vi "Write StateUART.vi"(8 "error in (no error)":errorcluster, 10 "STATEUART":T1, 11 "GiaoTiepUART in":refnum<class "GiaoTiepUART.lvclass">) -> (0 "error out":errorcluster, 3 "GiaoTiepUART out":refnum<class "GiaoTiepUART.lvclass">)   [LabVIEW 2014, in "LibraryGcode.lvlib" / "GiaoTiepUART.lvclass"]
uses:
  GiaoTiepUART.lvclass
  StateMachine_UART.ctl
  GiaoTiepUART.lvclass/GiaoTiepUART.ctl
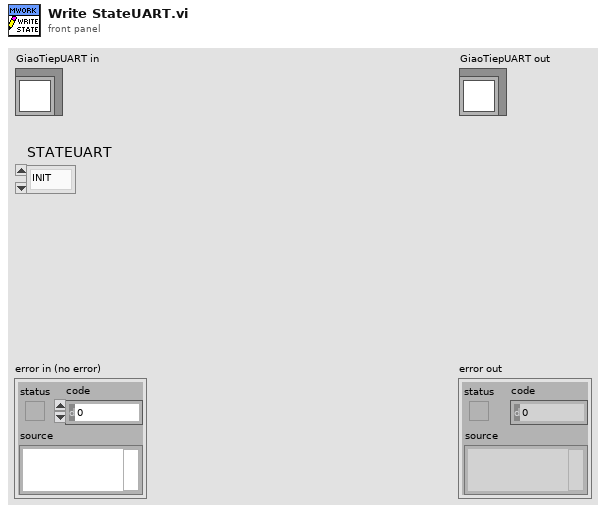
[diagram p1: front panel]
types:
  T1 = typedef "LibraryGcode.lvlib/GiaoTiepUART.lvclass/StateMachine_UART.ctl" = enum16{"INIT", "WRITE", "READ", "CHECKDATA", "IDLE", "STOP"}
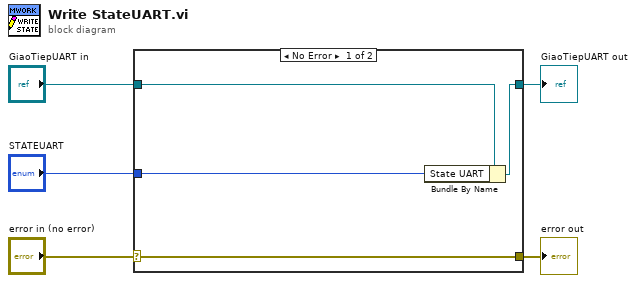
[diagram p0: block diagram]
diagram:
  n1 = case shown="No Error" "error in (no error)" {
    selector: "error in (no error)" -> [w9 w10]
    tunnel: [w9 w10] -> w4
    tunnel: [w8 w11] -> w2
    tunnel: "GiaoTiepUART in" -> [w6 w11]
    tunnel: "STATEUART" -> [w7 _]
    frame No Error {
      n2 = Bundle By Name(cluster=w6, "State UART"=w7) -> (w8:refnum<class "GiaoTiepUART.lvclass">)
    }
    frame Error {
    }
  }
  "error out" <- w4
  "GiaoTiepUART out" <- w2
